vi "Update TE MCLB.vi"(7 "TimingEngine":T1, 8 "error in":errorcluster, 9 "Selected Row":i32, 10 "Item Names":string[][](array[string]), 11 "FP Ctrls":refnum<class "FP Controls.lvclass">) -> (0 "error out":errorcluster, 3 "FP Ctrls":refnum<class "FP Controls.lvclass">)   [LabVIEW 2012, in "Configuration Grandmaster.lvlib" / "FP Controls.lvclass"]
uses:
  FP Controls.lvclass
  Common/Controls/TE_Designator.ctl
  FP Controls.lvclass/FP Controls.ctl
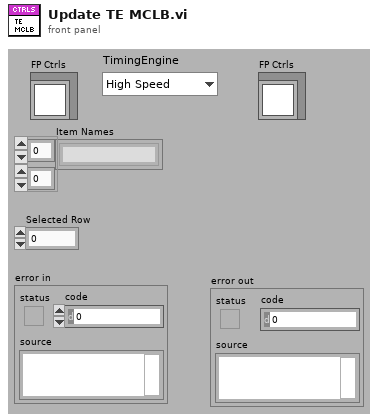
[diagram p1: front panel]
types:
  T1 = typedef "TE_Designator.ctl" = enum16{"High Speed", "Low Speed"}
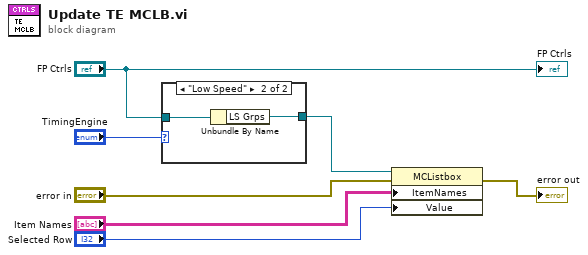
[diagram p0: block diagram]
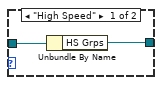
[diagram p2: hidden frame]
diagram:
  n1 = case shown="\"Low Speed\"" "TimingEngine" {
    tunnel: "FP Ctrls" -> [w9 w11]
    tunnel: [w8 w10] -> w2
    frame "High Speed" {
      n2 = Unbundle By Name(w9) -> ("HS Grps"=w8:refnum<vi>)
    }
    frame "Low Speed" {
      n3 = Unbundle By Name(w11) -> ("LS Grps"=w10:refnum<vi>)
    }
  }
  n4 = property on="Property Node" class="MCListbox"(reference=w2, error in="error in", "ItemNames"="Item Names", "Value"="Selected Row") -> (error out=→"error out":errorcluster)  [unwired: 1 out]
  "FP Ctrls" <- "FP Ctrls"
